vi "WaveformGraph_Filtros.vi"() -> ()   [LabVIEW 2022 SP3]
uses:
  <vilib>/express/express analysis/Spectral/Block/exnSpectralBlock spectral measurements RMS poly.vi
  <vilib>/express/express analysis/Spectral/Block/exnSpectralBlock spectral measurements RMS DDT.vi
  <vilib>/express/express analysis/Spectral/XNode/ExpressSpectralMeasurementsBlockNode.xnode
  <vilib>/measure/NI_MABase.lvlib
panel:
  in  "stop":bool
  out "Frequency Response":dynamicdata(graph)
  out "Time Response":dynamicdata(graph)
  out "Vp":dbl
  out "Vpp":dbl
  out "RMS Value":dbl
  in  "Cut Frequency":dbl
  in  "Off-set":dbl
  in  "Phase":dbl
  in  "Frequency":dbl
  in  "Amplitude":dbl
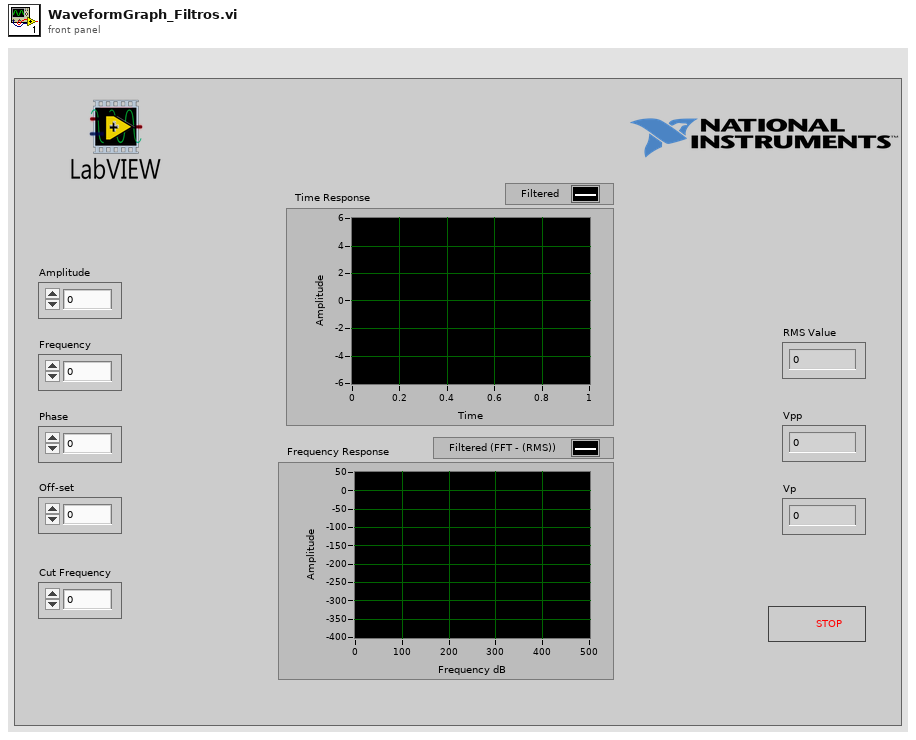
[diagram p1: front panel]
types:
  T1 = cluster{"averaging mode":u16, "weighting mode":u16, "number of averages":u32}
  T2 = cluster{"dB On (F)":bool, "unwrap phase (F)":bool, "convert to degree (F)":bool}
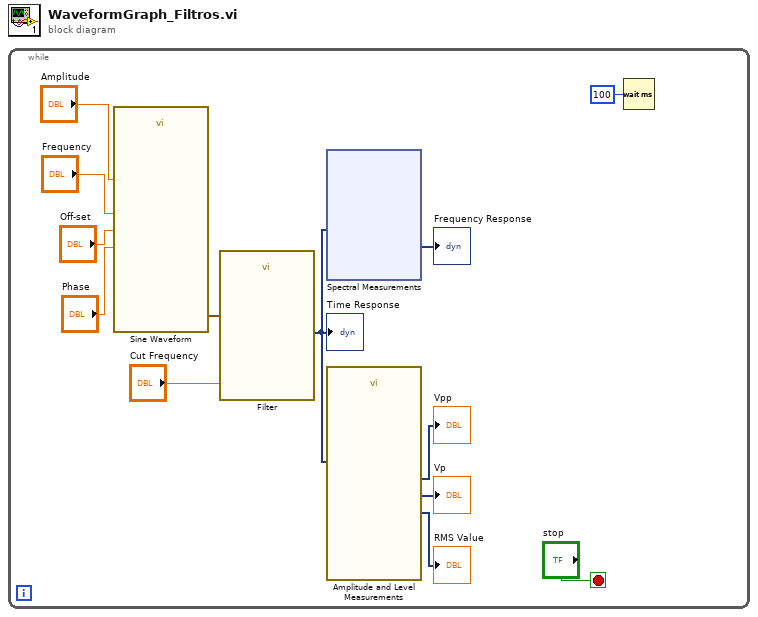
[diagram p0: block diagram]
diagram:
  n1 = while {
    stop <- "stop" stop-if-true
    n2 = call <vilib>:"Sine Waveform.vi"("offset"="Off-set", "phase"="Phase", "amplitude"="Amplitude", "frequency"="Frequency") -> ("signal out"=w8:waveform(dbl))  [unwired: 6 in, 1 out]
    n3 = call "Filter"("Lower Cut-Off"="Cut Frequency", "Signal"=w8) -> ("Filtered Signal"=w3:dynamicdata)  [unwired: 8 in, 1 out]
    "Time Response" <- w3
    n4 = xnode "Spectral Measurements"("Signals"=w3) -> ("FFT - (RMS)"=→"Frequency Response":dynamicdata)  [unwired: 1 in, 2 out]
    n5 = call "Amplitude and Level Measurements"("Signals"=w3) -> ("RMS"=→"RMS Value":dynamicdata, "Positive Peak"=→"Vp":dynamicdata, "Peak to Peak"=→"Vpp":dynamicdata)  [unwired: 11 in, 1 out]
    n6 = Wait (ms)(milliseconds to wait=u32 100) -> ()  [unwired: 1 out]
  }
